vi "DMA.Create Transfer (Scatter-Gather).vi"(8 "error in (no error)":errorcluster, 9 "RFM Offset":u32 format="%08x", 10 "Block Descriptors":T2[](array[typedef]) {"next descriptor ptr" format="%08x"; "data size" format="%08x"; "data ptr (upper)" format="%08x"; "data ptr (lower)" format="%08x"; "descriptor ptr (aligned)" format="%08x"; "descriptor size" format="%08x"; "descriptor ptr (VISA)" format="%08x"}, 11 "GE 5565PIORC in":refnum<class "GE 5565PIORC.lvclass">) -> (0 "error out":errorcluster, 1 "Transfer Size (bytes)":u32, 2 "Scatter-Gather Transfer Spec":T1 {"Block Descriptors"."next descriptor ptr" format="%08x"; "Block Descriptors"."data size" format="%08x"; "Block Descriptors"."data ptr (upper)" format="%08x"; "Block Descriptors"."data ptr (lower)" format="%08x"; "Block Descriptors"."descriptor ptr (aligned)" format="%08x"; "Block Descriptors"."descriptor size" format="%08x"; "Block Descriptors"."descriptor ptr (VISA)" format="%08x"; "RFM Address" format="%08x"}, 3 "GE 5565PIORC out":refnum<class "GE 5565PIORC.lvclass">)   [LabVIEW 2016, in "GE 5565PIORC.lvclass"]
uses:
  GE 5565PIORC.lvclass
  Controls/DMA Block Descriptor.ctl
  Controls/DMA Transfer Spec (Scatter-Gather).ctl
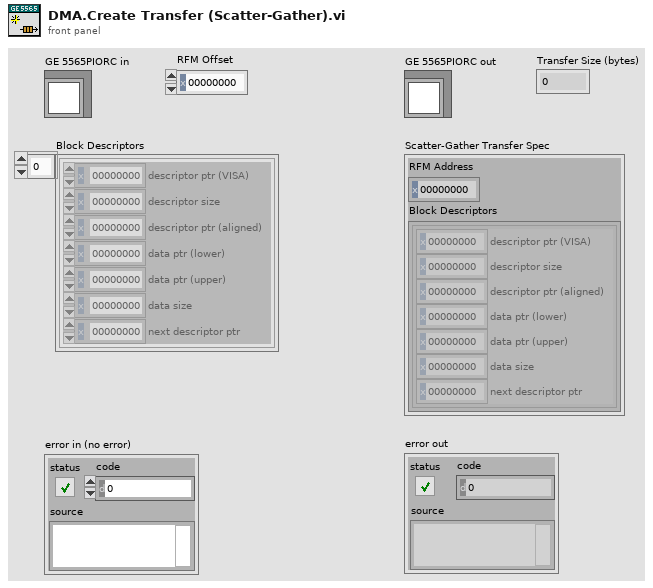
[diagram p1: front panel]
types:
  T1 = typedef "GE 5565PIORC.lvclass/DMA Transfer Spec (Scatter-Gather).ctl" = cluster{"RFM Address":u32, "Block Descriptors":T2[]}
  T2 = typedef "GE 5565PIORC.lvclass/DMA Block Descriptor.ctl" = cluster{"descriptor ptr (VISA)":u32, "descriptor size":u32, "descriptor ptr (aligned)":u32, "data ptr (lower)":u32, "data ptr (upper)":u32, "data size":u32, "next descriptor ptr":u32}
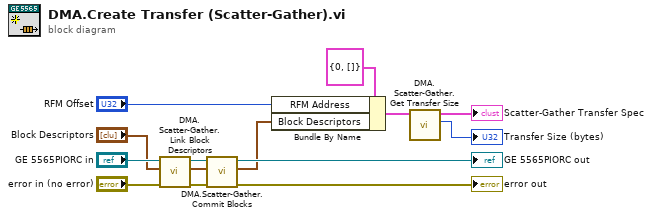
[diagram p0: block diagram]
diagram:
  n1 = call "DMA.Scatter-Gather.Link Block Descriptors.vi"("error in (no error)"="error in (no error)", "Block Descriptors"="Block Descriptors", "GE 5565PIORC in"="GE 5565PIORC in") -> ("error out"=w11:errorcluster, "Block Descriptors out"=w12:T2[], "GE 5565PIORC out"=w13:refnum<class "GE 5565PIORC.lvclass">)  [unwired: 6 in]
  n2 = call "DMA.Scatter-Gather.Commit Blocks.vi"("error in (no error)"=w11, "Block Descriptors"=w12, "GE 5565PIORC in"=w13) -> ("error out"=→"error out":errorcluster, "Block Descriptors out"=w5:T2[], "GE 5565PIORC out"=→"GE 5565PIORC out":refnum<class "GE 5565PIORC.lvclass">)  [unwired: 6 in]
  n3 = Bundle By Name(cluster=T1 {"RFM Address"=0, "Block Descriptors"=[]} ("Transfer Spec (Block)"), "RFM Address"="RFM Offset", "Block Descriptors"=w5) -> (w3:T1)
  n4 = call "DMA.Scatter-Gather.Get Transfer Size.vi"("Scatter-Gather Transfer Spec"=w3) -> ("Transfer Size (bytes)"=→"Transfer Size (bytes)":u32, "Scatter-Gather Transfer Spec out"=→"Scatter-Gather Transfer Spec":T1)  [unwired: 9 in]
